vi "Lakeshore_372_write.vi"(5 "File reference":refnum<file>) -> ()   [LabVIEW 2016]
uses:
  Instrument_Setup.vi
  Global/Global Variables/global.vi
  Global/Global Variables/Data_Display_global.vi
panel:
  # "OFF"
  # "ON"
  # "OFF"
  # "ON"
  # "OFF"
  # "ON"
  # "OFF"
  # "ON"
  # "ON"
  # "OFF"
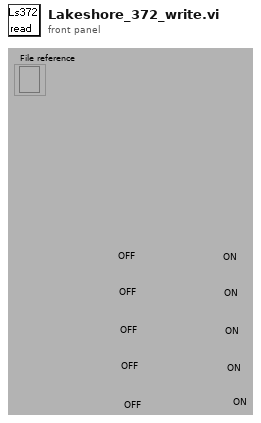
[diagram p1: front panel]
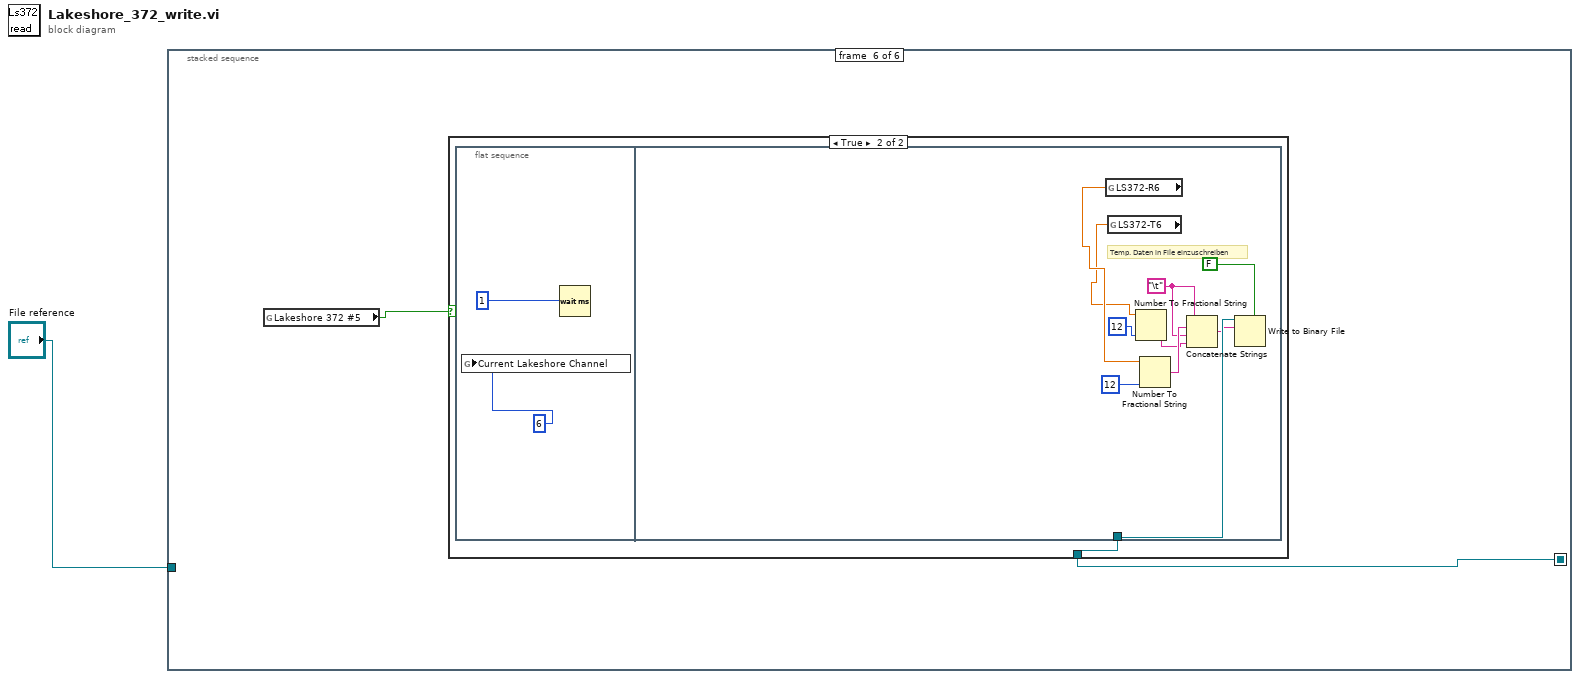
[diagram p0: block diagram]
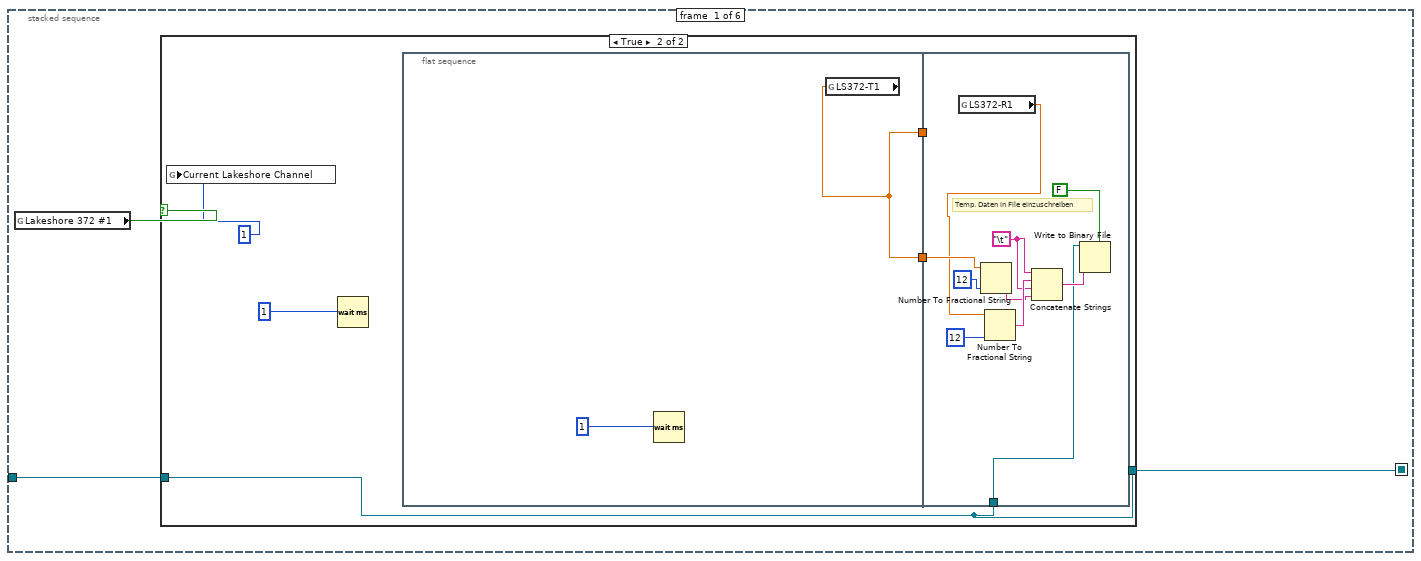
[diagram p2: hidden frame]
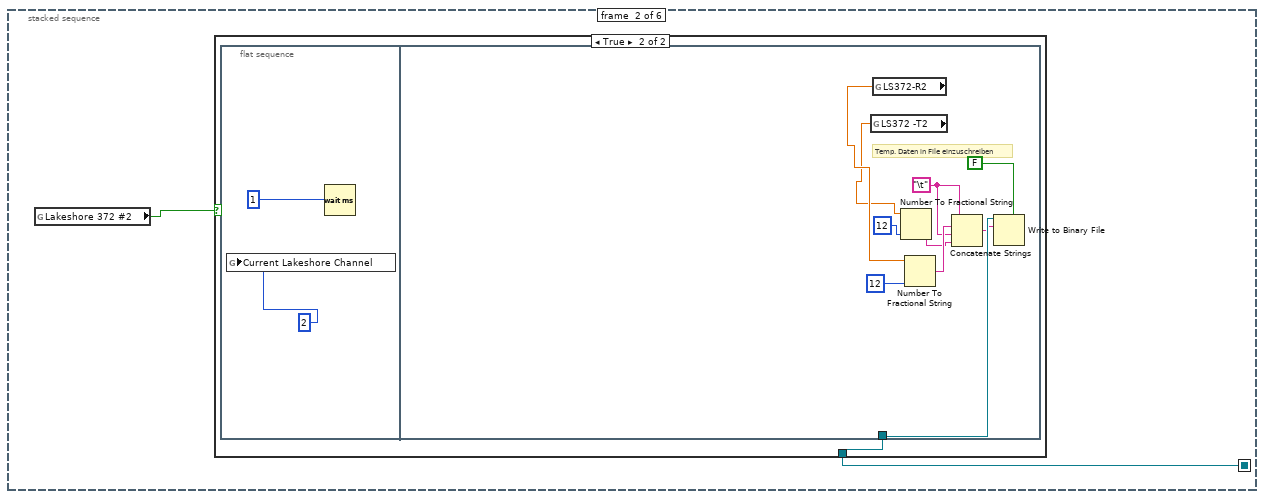
[diagram p4: hidden frame]
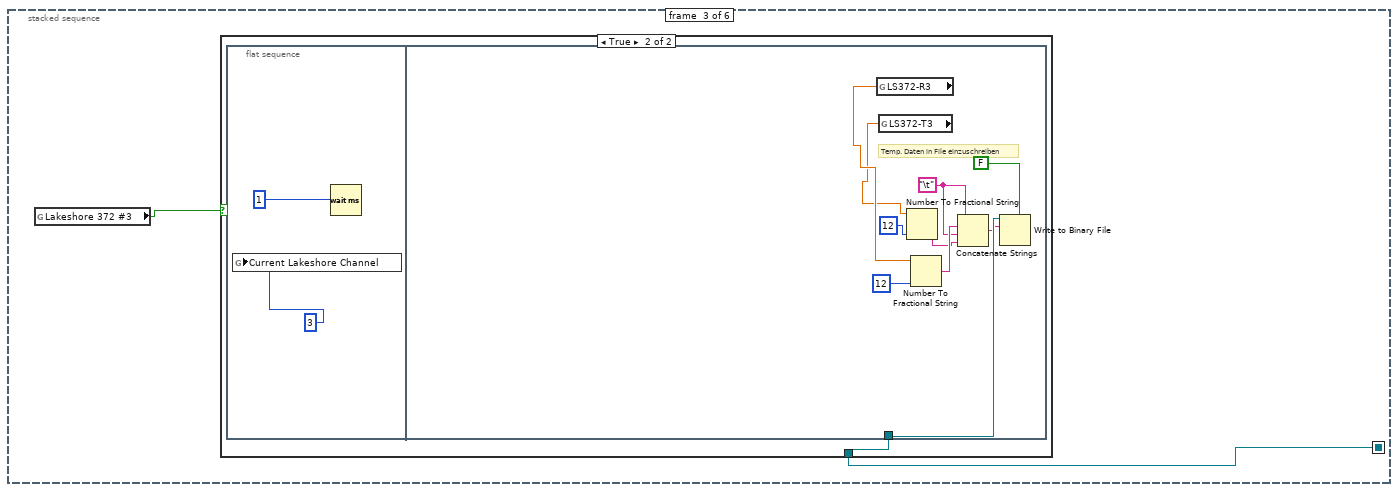
[diagram p6: hidden frame]
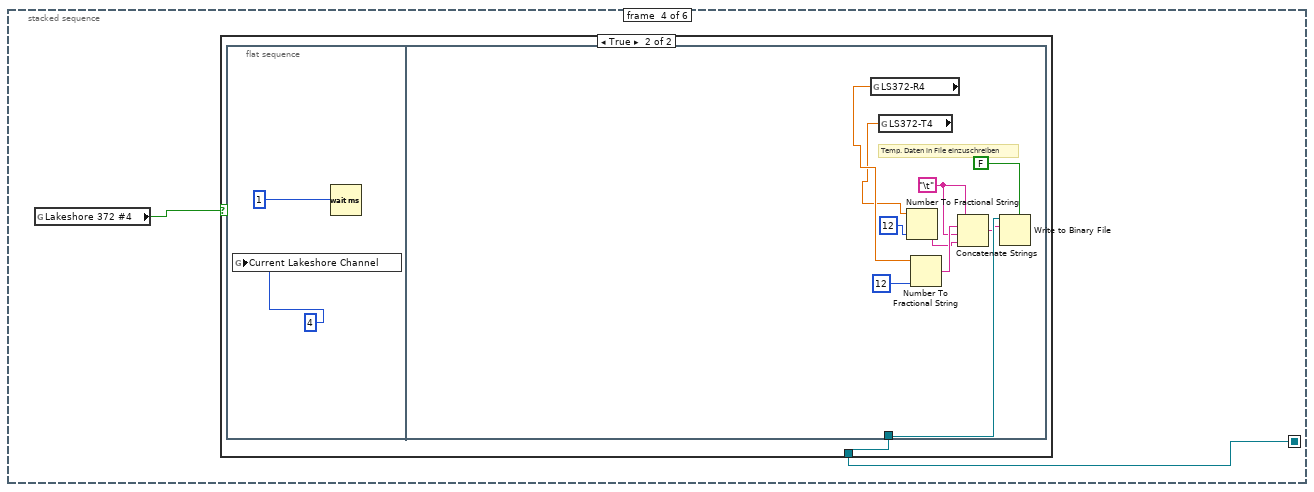
[diagram p8: hidden frame]
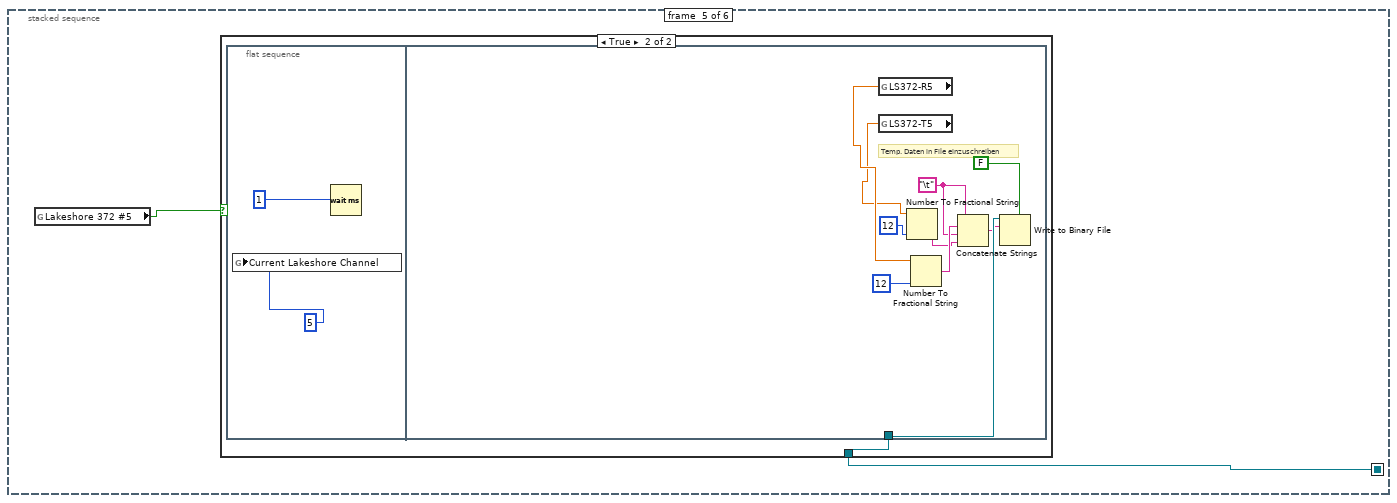
[diagram p10: hidden frame]
diagram:
  n1 = stacked-sequence {
    seq-local: [w2 _ _ _ _ _] -> [_ w23 w38 w53 w68 w83]
    tunnel: "File reference" -> [w3 _ _ _ _ _]
    frame #0 {
      n2 = global read "Instrument_Setup.vi" "Lakeshore 372 #1"() -> (w4:bool)
      n3 = case shown="True" w4 {
        tunnel: w3 -> [w5 w10]
        tunnel: [w5 w10] -> w2
        frame False {
        }
        frame True {
          n4 = global write "global.vi" "Current Lakeshore Channel"(1) -> ()
          n5 = Wait (ms)(milliseconds to wait=1) -> ()  [unwired: 1 out]
          n6 = flat-sequence {
            tunnel: [w11] -> w9
            tunnel: [w11] -> w7
            tunnel: w10 -> [w18]
            tunnel: w9 -> [w16]
            tunnel: w7 -> [_]
            frame #0 {
              n7 = Wait (ms)(milliseconds to wait=1) -> ()  [unwired: 1 out]
              n8 = global read "Data_Display_global.vi" "LS372-T1"() -> (w11:dbl)
            }
            frame #1 {
              w15 = "\t"
              # "Temp. Daten in File einzuschreiben"
              n9 = global read "Data_Display_global.vi" "LS372-R1"() -> (w13:dbl)
              n10 = Number To Fractional String(number=w16, precision (6)=i16 12) -> (F-format string=w14:string)  [unwired: 2 in]
              n11 = Number To Fractional String(number=w13, precision (6)=i16 12) -> (F-format string=w21:string)  [unwired: 2 in]
              n12 = Concatenate Strings(w15, w21, w15, w14) -> (w22:string)
              n13 = Write to Binary File ("Write File")(file (use dialog)=w18, data=w22, 5:FALSE ("prepend array or string size? (T)")) -> ()  [unwired: 3 in, 3 out]
            }
          }
        }
      }
    }
    frame #1 {
      n14 = global read "Instrument_Setup.vi" "Lakeshore 372 #2"() -> (w24:bool)
      n15 = case shown="True" w24 {
        tunnel: w23 -> [_ w25]
        frame False {
        }
        frame True {
          n16 = flat-sequence {
            tunnel: w25 -> [w36]
            frame #0 {
              n17 = global write "global.vi" "Current Lakeshore Channel"(2) -> ()
              n18 = Wait (ms)(milliseconds to wait=1) -> ()  [unwired: 1 out]
            }
            frame #1 {
              w32 = "\t"
              # "Temp. Daten in File einzuschreiben"
              n19 = global read "Data_Display_global.vi" "LS372 -T2"() -> (w28:dbl)
              n20 = global read "Data_Display_global.vi" "LS372-R2"() -> (w29:dbl)
              n21 = Number To Fractional String(number=w28, precision (6)=i16 12) -> (F-format string=w31:string)  [unwired: 2 in]
              n22 = Number To Fractional String(number=w29, precision (6)=i16 12) -> (F-format string=w35:string)  [unwired: 2 in]
              n23 = Concatenate Strings(w32, w35, w32, w31) -> (w30:string)
              n24 = Write to Binary File ("Write File")(file (use dialog)=w36, data=w30, 5:FALSE ("prepend array or string size? (T)")) -> ()  [unwired: 3 in, 3 out]
            }
          }
        }
      }
    }
    frame #2 {
      n25 = global read "Instrument_Setup.vi" "Lakeshore 372 #3"() -> (w39:bool)
      n26 = case shown="True" w39 {
        tunnel: w38 -> [_ w40]
        frame False {
        }
        frame True {
          n27 = flat-sequence {
            tunnel: w40 -> [w51]
            frame #0 {
              n28 = global write "global.vi" "Current Lakeshore Channel"(3) -> ()
              n29 = Wait (ms)(milliseconds to wait=1) -> ()  [unwired: 1 out]
            }
            frame #1 {
              w47 = "\t"
              # "Temp. Daten in File einzuschreiben"
              n30 = global read "Data_Display_global.vi" "LS372-R3"() -> (w44:dbl)
              n31 = global read "Data_Display_global.vi" "LS372-T3"() -> (w43:dbl)
              n32 = Number To Fractional String(number=w43, precision (6)=i16 12) -> (F-format string=w46:string)  [unwired: 2 in]
              n33 = Number To Fractional String(number=w44, precision (6)=i16 12) -> (F-format string=w50:string)  [unwired: 2 in]
              n34 = Concatenate Strings(w47, w50, w47, w46) -> (w45:string)
              n35 = Write to Binary File ("Write File")(file (use dialog)=w51, data=w45, 5:FALSE ("prepend array or string size? (T)")) -> ()  [unwired: 3 in, 3 out]
            }
          }
        }
      }
    }
    frame #3 {
      n36 = global read "Instrument_Setup.vi" "Lakeshore 372 #4"() -> (w54:bool)
      n37 = case shown="True" w54 {
        tunnel: w53 -> [_ w55]
        frame False {
        }
        frame True {
          n38 = flat-sequence {
            tunnel: w55 -> [w66]
            frame #0 {
              n39 = global write "global.vi" "Current Lakeshore Channel"(4) -> ()
              n40 = Wait (ms)(milliseconds to wait=1) -> ()  [unwired: 1 out]
            }
            frame #1 {
              w62 = "\t"
              # "Temp. Daten in File einzuschreiben"
              n41 = global read "Data_Display_global.vi" "LS372-R4"() -> (w59:dbl)
              n42 = global read "Data_Display_global.vi" "LS372-T4"() -> (w58:dbl)
              n43 = Number To Fractional String(number=w58, precision (6)=i16 12) -> (F-format string=w61:string)  [unwired: 2 in]
              n44 = Number To Fractional String(number=w59, precision (6)=i16 12) -> (F-format string=w65:string)  [unwired: 2 in]
              n45 = Concatenate Strings(w62, w65, w62, w61) -> (w60:string)
              n46 = Write to Binary File ("Write File")(file (use dialog)=w66, data=w60, 5:FALSE ("prepend array or string size? (T)")) -> ()  [unwired: 3 in, 3 out]
            }
          }
        }
      }
    }
    frame #4 {
      n47 = global read "Instrument_Setup.vi" "Lakeshore 372 #5"() -> (w69:bool)
      n48 = case shown="True" w69 {
        tunnel: w68 -> [_ w70]
        frame False {
        }
        frame True {
          n49 = flat-sequence {
            tunnel: w70 -> [w81]
            frame #0 {
              n50 = global write "global.vi" "Current Lakeshore Channel"(5) -> ()
              n51 = Wait (ms)(milliseconds to wait=1) -> ()  [unwired: 1 out]
            }
            frame #1 {
              w77 = "\t"
              # "Temp. Daten in File einzuschreiben"
              n52 = global read "Data_Display_global.vi" "LS372-R5"() -> (w74:dbl)
              n53 = global read "Data_Display_global.vi" "LS372-T5"() -> (w73:dbl)
              n54 = Number To Fractional String(number=w73, precision (6)=i16 12) -> (F-format string=w76:string)  [unwired: 2 in]
              n55 = Number To Fractional String(number=w74, precision (6)=i16 12) -> (F-format string=w80:string)  [unwired: 2 in]
              n56 = Concatenate Strings(w77, w80, w77, w76) -> (w75:string)
              n57 = Write to Binary File ("Write File")(file (use dialog)=w81, data=w75, 5:FALSE ("prepend array or string size? (T)")) -> ()  [unwired: 3 in, 3 out]
            }
          }
        }
      }
    }
    frame #5 {
      n58 = global read "Instrument_Setup.vi" "Lakeshore 372 #5"() -> (w84:bool)
      n59 = case shown="True" w84 {
        tunnel: w83 -> [_ w85]
        frame False {
        }
        frame True {
          n60 = flat-sequence {
            tunnel: w85 -> [w96]
            frame #0 {
              n61 = global write "global.vi" "Current Lakeshore Channel"(6) -> ()
              n62 = Wait (ms)(milliseconds to wait=1) -> ()  [unwired: 1 out]
            }
            frame #1 {
              w92 = "\t"
              # "Temp. Daten in File einzuschreiben"
              n63 = global read "Data_Display_global.vi" "LS372-R6"() -> (w89:dbl)
              n64 = global read "Data_Display_global.vi" "LS372-T6"() -> (w88:dbl)
              n65 = Number To Fractional String(number=w88, precision (6)=i16 12) -> (F-format string=w91:string)  [unwired: 2 in]
              n66 = Number To Fractional String(number=w89, precision (6)=i16 12) -> (F-format string=w95:string)  [unwired: 2 in]
              n67 = Concatenate Strings(w92, w95, w92, w91) -> (w90:string)
              n68 = Write to Binary File ("Write File")(file (use dialog)=w96, data=w90, 5:FALSE ("prepend array or string size? (T)")) -> ()  [unwired: 3 in, 3 out]
            }
          }
        }
      }
    }
  }
